vi "Create Standard Waveform.vi"(11 "Suggested Sample Rate (Hz)":dbl=10000000.0 min=0.0 format="%#_6p") -> (2 "Waveform Created?":bool, 3 "Output Waveform":waveform(dbl))   [LabVIEW 2025, in "TDMS Waveform Creator UI.lvlib"]
uses:
  TDMS Waveform Creator UI.lvlib
panel:
  in  "Post Delay (s)":dbl min=0.0 format="%#_6p"
  in  "Pre Delay (s)":dbl min=0.0 format="%#_6p"
  out "Waveform Name":string
  in  "Cancel":bool
  in  "OK":bool
  out "Actual Sample Size":i32
  out "Actual Duration (s)":dbl format="%#_6p"
  out "Waveform Preview":waveform(dbl)(graph)
  in  "Sample Rate (Hz)":dbl=10000000.0 min=0.0 format="%#_6p"
  in  "Config Type":enum32{"Periodic", "Ramp", "DC"}(tab)
  in  "Number of Cycles":u32=1 min=1
  in  "Frequency (Hz)":dbl=10000.0 format="%#_6p"
  in  "Amplitude":dbl=1.0
  in  "Ramp Start":dbl
  in  "Ramp Stop":dbl=1.0
  in  "Length (s)":dbl=0.001 format="%#_6p"
  in  "DC Value":dbl format="%#_6p"
  in  "Duration (s)":dbl=0.001 format="%#_6p"
  in  "Waveform Type":i32(listbox)
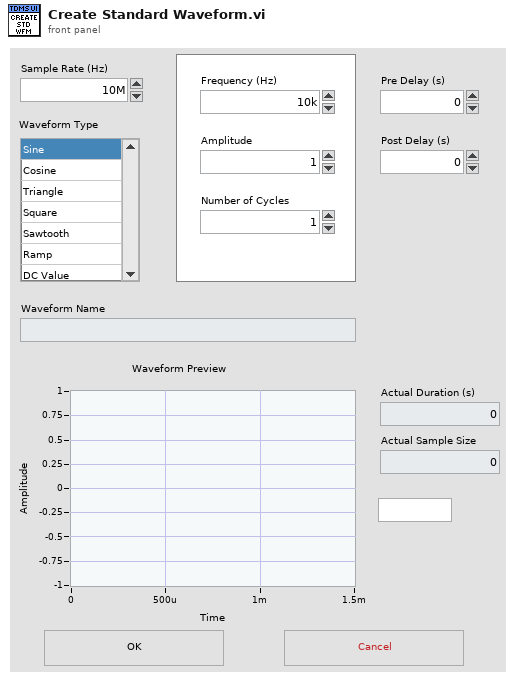
[diagram p1: front panel]
types:
  T1 = cluster{"Waveform Type":i32, "Sample Rate (Hz)":dbl, "Frequency (Hz)":dbl, "Amplitude":dbl, "Number of Cycles":u32, "Ramp Start":dbl, "Ramp Stop":dbl, "Length (s)":dbl, "DC Value":dbl, "Duration (s)":dbl, "Pre Delay (s)":dbl, "Post Delay (s)":dbl}
  T2 = enum8{"Enabled", "Disabled", "Disabled and Grayed Out"}
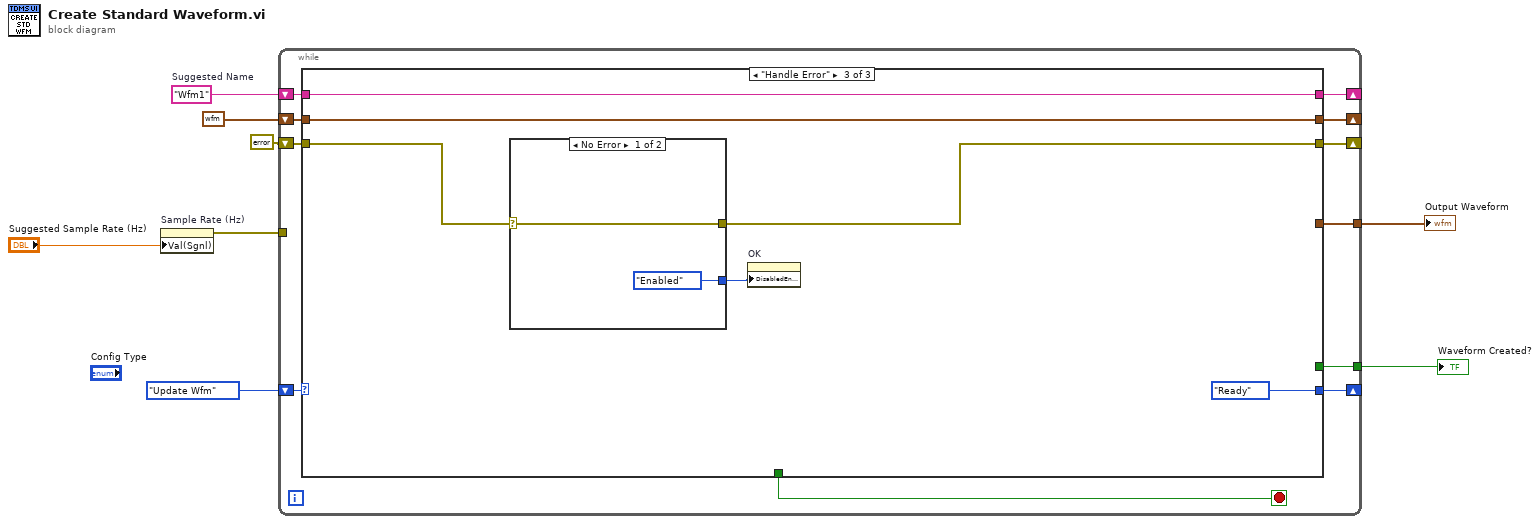
[diagram p0: block diagram]
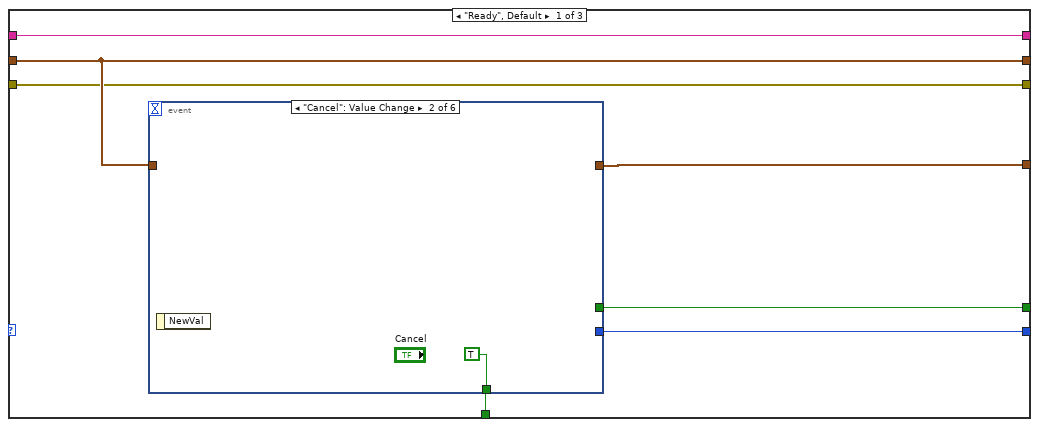
[diagram p2: hidden frame]
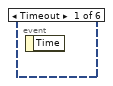
[diagram p3: hidden frame]
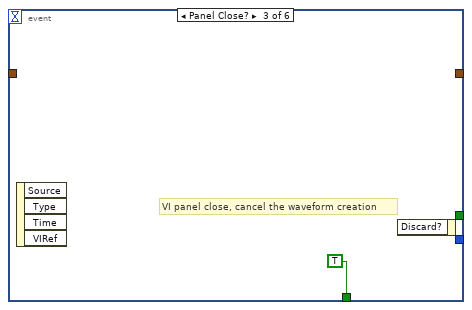
[diagram p4: hidden frame]
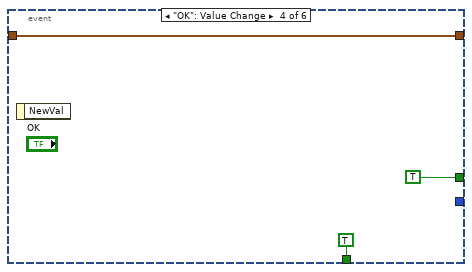
[diagram p5: hidden frame]
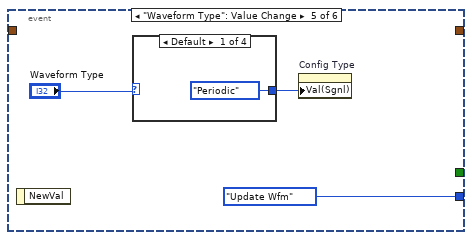
[diagram p6: hidden frame]
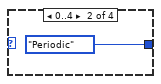
[diagram p7: hidden frame]
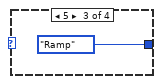
[diagram p8: hidden frame]
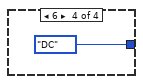
[diagram p9: hidden frame]
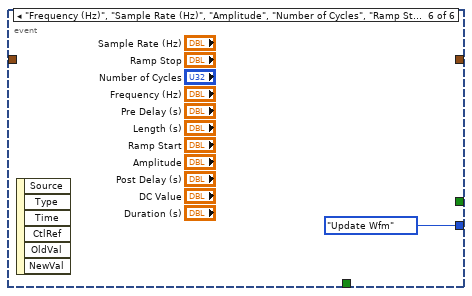
[diagram p10: hidden frame]
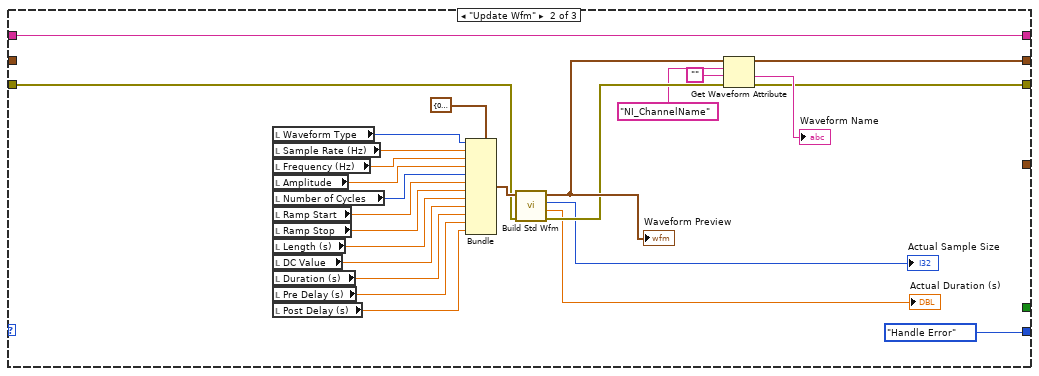
[diagram p11: hidden frame]
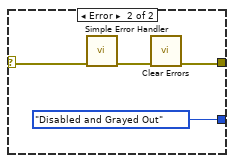
[diagram p12: hidden frame]
diagram:
  w6 = "Wfm1"  # Suggested Name
  n1 = property on="Sample Rate (Hz)" class="DigNum (strict)"("Val(Sgnl)"="Suggested Sample Rate (Hz)") -> (error out=w2:errorcluster)  [unwired: 2 in, 1 out]
  n2 = while {
    tunnel: [w18] -> w8
    shift-right: [w16] -> _
    shift-left: enum16{"Ready", "Update Wfm", "Handle Error"}."Update Wfm" -> [w17]
    shift-right: [w14] -> _
    shift-left: w6 -> [w15]
    shift-right: [w12] -> _
    shift-left: waveform(dbl) {"t0"=timestamp(0 s since 1904-01-01), "dt"=1.0, "Y"=[]} ("Output Waveform") -> [w13]
    tunnel: [w11] -> w4
    tunnel: w2 -> [_]
    shift-right: [w10] -> _
    shift-left: errorcluster {"status"=FALSE, "code"=0, "source"=""} ("error out") -> [w9]
    stop <- w19 stop-if-true
    n3 = case shown="\"Handle Error\"" w17 {
      tunnel: [w26 _ _] -> w19
      tunnel: [w25 _ _] -> w18
      tunnel: [w24 enum16{"Ready", "Update Wfm", "Handle Error"}."Handle Error" enum16{"Ready", "Update Wfm", "Handle Error"}."Ready"] -> w16
      tunnel: w15 -> [w23 w51 w70]
      tunnel: [w23 w51 w70] -> w14
      tunnel: w13 -> [w22 _ w71]
      tunnel: [w22 w50 w71] -> w12
      tunnel: [w21 _ _] -> w11
      tunnel: [w20 w45 w68] -> w10
      tunnel: w9 -> [w20 w44 w69]
      frame "Ready", Default {
        n4 = event shown="[1] \"Cancel\": Value Change" {
          selector: _ -> [_ _ _ _ _ _]
          dyn-events: _ -> [_ _ _ _ _ _]
          timeout: _ -> [_ _ _ _ _ _]
          tunnel: [_ TRUE TRUE TRUE _ _] -> w26
          tunnel: [_ _ _ TRUE _ _] -> w25
          tunnel: [_ _ _ _ enum16{"Ready", "Update Wfm", "Handle Error"}."Update Wfm" enum16{"Ready", "Update Wfm", "Handle Error"}."Update Wfm"] -> w24
          tunnel: w22 -> [_ _ _ w29 _ _]
          tunnel: [_ _ _ w29 _ _] -> w21
          event Timeout {
            n5 = event-data() -> ()  [unwired: 1 in, 1 out]
          }
          event "Cancel": Value Change {
            n6 = event-data() -> ()  [unwired: 1 in, 1 out]
          }
          event Panel Close? {
            # "VI panel close, cancel the waveform creation"
            n7 = event-data() -> ()  [unwired: 1 in, 4 out]
            n8 = event-data() -> ()  [unwired: 2 in, 1 out]
          }
          event "OK": Value Change {
            n9 = event-data() -> ()  [unwired: 1 in, 1 out]
          }
          event "Waveform Type": Value Change {
            n10 = event-data() -> ()  [unwired: 1 in, 1 out]
            n11 = case shown="Default" "Waveform Type" {
              tunnel: [enum32{"Periodic", "Ramp", "DC"}."Periodic" ("Value (Signaling)") enum32{"Periodic", "Ramp", "DC"}."Periodic" ("Value (Signaling)") enum32{"Periodic", "Ramp", "DC"}."Ramp" ("Value (Signaling)") enum32{"Periodic", "Ramp", "DC"}."DC" ("Value (Signaling)")] -> w34
              frame Default {
              }
              frame 0..4 {
              }
              frame 5 {
              }
              frame 6 {
              }
            }
            n12 = property on="Config Type" class="TabCtl (strict)"("Val(Sgnl)"=w34) -> ()  [unwired: 2 in, 2 out]
          }
          event "Frequency (Hz)", "Sample Rate (Hz)", "Amplitude", "Number of Cycles", "Ramp Start", "Ramp Stop", "Length (s)", "Duration (s)", "DC Value", "Pre Delay (s)", "Post Delay (s)": Value Change {
            n13 = event-data() -> ()  [unwired: 1 in, 6 out]
          }
        }
      }
      frame "Update Wfm" {
        n14 = local read "Waveform Type"() -> (w41:i32)
        n15 = local read "Sample Rate (Hz)"() -> (w65:dbl)
        n16 = local read "Frequency (Hz)"() -> (w64:dbl)
        n17 = local read "Amplitude"() -> (w63:dbl)
        n18 = local read "Number of Cycles"() -> (w62:u32)
        n19 = local read "Ramp Start"() -> (w61:dbl)
        n20 = local read "Ramp Stop"() -> (w60:dbl)
        n21 = local read "Length (s)"() -> (w59:dbl)
        n22 = local read "DC Value"() -> (w58:dbl)
        n23 = local read "Duration (s)"() -> (w57:dbl)
        n24 = local read "Pre Delay (s)"() -> (w56:dbl)
        n25 = local read "Post Delay (s)"() -> (w55:dbl)
        n26 = Bundle(cluster=T1 {"Waveform Type"=0, "Sample Rate (Hz)"=10000000.0, "Frequency (Hz)"=2000.0, "Amplitude"=1.0, "Number of Cycles"=1, "Ramp Start"=0.0, "Ramp Stop"=1.0, "Length (s)"=0.001, "DC Value"=0.0, "Duration (s)"=0.001, "Pre Delay (s)"=0.0, "Post Delay (s)"=0.0} ("Standard Wfm Config"), "Waveform Type"=w41, "Sample Rate (Hz)"=w65, "Frequency (Hz)"=w64, "Amplitude"=w63, "Number of Cycles"=w62, "Ramp Start"=w61, "Ramp Stop"=w60, "Length (s)"=w59, "DC Value"=w58, "Duration (s)"=w57, "Pre Delay (s)"=w56, "Post Delay (s)"=w55) -> (w54:T1)
        n27 = call "Build Std Wfm.vi"("error in"=w44, "Standard Wfm Config"=w54) -> ("error out"=w49:errorcluster, "Actual Duration (s)"=→"Actual Duration (s)":dbl, "Actual Sample Size"=→"Actual Sample Size":i32, "Waveform"=w52:waveform(dbl))  [unwired: 6 in]
        "Waveform Preview" <- w52
        n28 = Get Waveform Attribute(4:w49, 5:"", 6:"NI_ChannelName" ("name"), 7:w52) -> (0:w45:errorcluster, 1:→"Waveform Name":string, 3:w50:waveform(dbl))  [unwired: 1 out]
      }
      frame "Handle Error" {
        n29 = case shown="No Error" w69 {
          selector: w69 -> [w73 w77]
          tunnel: [w73 w74] -> w68
          tunnel: [T2."Enabled" ("DisabledEnum") T2."Disabled and Grayed Out" ("DisabledEnum")] -> w67
          frame No Error {
          }
          frame Error {
            n30 = call <vilib>:"Simple Error Handler.vi"("error in (no error)"=w77) -> ("error out"=w76:errorcluster)  [unwired: 4 in, 4 out]
            n31 = call <vilib>:"Clear Errors.vi"("error in (no error)"=w76) -> ("error out"=w74:errorcluster)  [unwired: 5 in, 1 out]
          }
        }
        n32 = property on="OK" class="Bool"("DisabledEnum"=w67) -> ()  [unwired: 2 in, 2 out]
      }
    }
  }
  "Waveform Created?" <- w8
  "Output Waveform" <- w4
